vi "S30c_dll F30.vi"(4 "error in":errorcluster, 6 "Nr.":u8=64, 7 "Dev Addr":u8=250) -> (0 "error out":errorcluster, 2 "Coefficient":sgl format="%_6e")   [LabVIEW 2014, in "K_S30c_dll.lvlib"]
uses:
  K_S30c_dll.lvlib
  s30c.dll
panel:
  # "Function 30: Read coefficient\n\nusing s30c.dll\nKeller AG für Druckmesstechnik, 29.5.08 b.v."
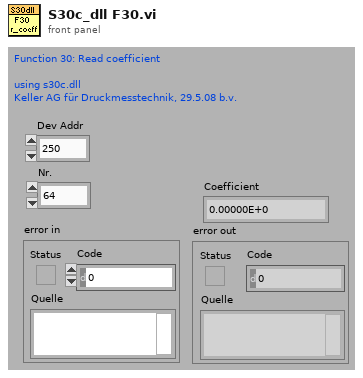
[diagram p1: front panel]
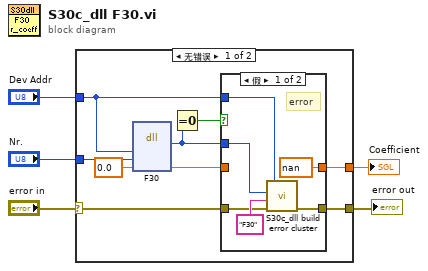
[diagram p0: block diagram]
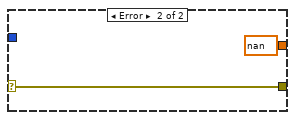
[diagram p3: hidden frame]
diagram:
  n1 = case shown="无错误" "error in" {
    selector: "error in" -> [w12 w23]
    tunnel: [w13 w23] -> w3
    tunnel: "Dev Addr" -> [w9 _]
    tunnel: [w11 sgl nan ("Coeff")] -> w4
    tunnel: "Nr." -> [w8 _]
    frame No Error {
      n2 = dll-call lib="PTH2Labs EworkSINOPEC北控自动相渗software2.08.5_dlls30c.dll" fn="F30"("DevAddr"=w9, "Coeff No"=w8, "Coeff"=sgl 0.0) -> (w7:i16, "Coeff"=w6:sgl)  [unwired: 5 in, 2 out]
      n3 = Equal To 0?(x=w7) -> (x = 0?=w14:bool)
      n4 = case shown="假" w14 {
        tunnel: [w20 w21] -> w13
        tunnel: w7 -> [w18 _]
        tunnel: w9 -> [w19 _]
        tunnel: w12 -> [w16 w21]
        tunnel: w6 -> [_ w22]
        tunnel: [sgl nan ("Coeff") w22] -> w11
        frame False {
          # "error"
          n5 = call "S30c_dll build error cluster.vi"("error in"=w16, "error Text"="F30", "error code"=w18, "Dev Addr"=w19) -> ("error out"=w20:errorcluster)  [unwired: 3 in]
        }
        frame True {
        }
      }
    }
    frame Error {
    }
  }
  "error out" <- w3
  "Coefficient" <- w4
